vi "at Max velocity.vi"(8 "error in (no error) 2":errorcluster, 9 "Previous Velocity 2":i32, 10 "Previous Velocity":i32) -> (0 "error out 2":errorcluster, 1 "New Velocity 2":i32, 2 "New Velocity":i32, 3 "Max Velocity":bool)   [LabVIEW 2017]
uses:
  Public/Documents/Cross The Road Electronics/Phoenix-LabVIEW/Motor Controller/Get/CTRE_Phoenix_MotorController_GetSelectedSensorData.vi
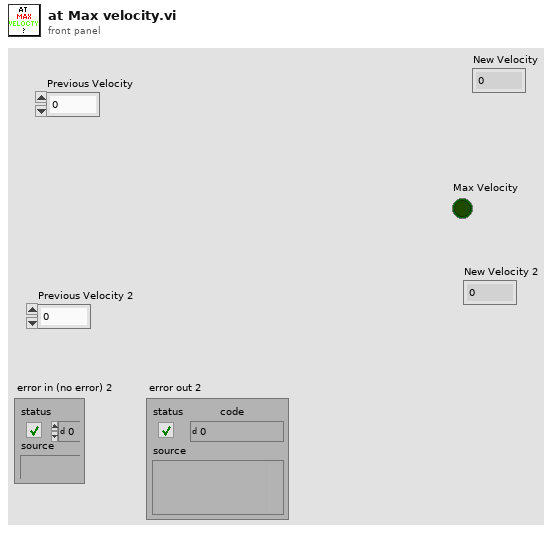
[diagram p1: front panel]
types:
  T1 = typedef "WPI_MotorControlDeviceRef.ctl" = cluster{"DeviceStatus":errorcluster, "Type":T2, "PWM":cluster{"PWM Channel":T3, "DeadBand":T4}, "CAN":cluster{"Device Number":u8, "SetOutput VI Ref":variant, "GetOutput VI Ref":variant, "Enable VI Ref":variant, "Disable VI Ref":variant, "Data":variant}, "Invert":bool, "DIO PWM":cluster{"PWM \"Enable\" Channel":T3, "DIOChannel":T5, "PWM Rate":dbl}}
  T2 = typedef "WPI_MotorControlType.ctl" = enum16{"PWM", "CAN", "DIO PWM"}
  T3 = typedef "FPGA_DIOPWMChannel.ctl" = enum8{"PWM 0", "PWM 1", "PWM 2", "PWM 3", "PWM 4", "PWM 5", "PWM 6", "PWM 7", "PWM 8", "PWM 9", "PWM MXP 0", "PWM MXP 1", "PWM MXP 2", "PWM MXP 3", "PWM MXP 4", "PWM MXP 5", "PWM MXP 6", "PWM MXP 7", "PWM MXP 8", "PWM MXP 9", "Invalid"}
  T4 = typedef "WPI_PWMDeadband.ctl" = cluster{"Name":string, "maxPositivePwm":i32, "minPositivePwm":i32, "centerPwm":i32, "maxNegativePwm":i32, "minNegativePwm":i32, "angularRange":u16}
  T5 = typedef "FPGA_DIOChannel.ctl" = enum8{"DIO 0", "DIO 1", "DIO 2", "DIO 3", "DIO 4", "DIO 5", "DIO 6", "DIO 7", "DIO 8", "DIO 9", "DIO MXP 0", "DIO MXP 1", "DIO MXP 2", "DIO MXP 3", "DIO MXP 4", "DIO MXP 5", "DIO MXP 6", "DIO MXP 7", "DIO MXP 8", "DIO MXP 9", "DIO MXP 10", "DIO MXP 11", "DIO MXP 12", "DIO MXP 13", "DIO MXP 14", "DIO MXP 15", "SPI Port CS1", "SPI Port CS2", "SPI Port CS3", "SPI Port MISO", "SPI Port MOSI", "Invalid"}
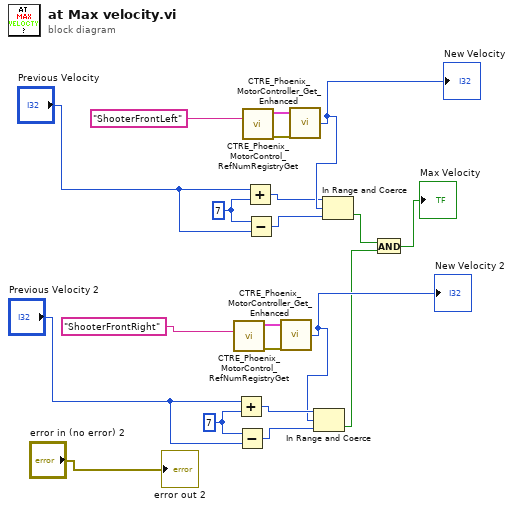
[diagram p0: block diagram]
diagram:
  w11 = 7
  w15 = 7
  n1 = call "CTRE_Phoenix_MotorControl_RefNumRegistryGet.vi"("refnum name"="ShooterFrontRight") -> ("error out"=w6:errorcluster, "PhoenixMotorControlDevRef"=w7:T1)  [unwired: 9 in]
  n2 = Add(x="Previous Velocity 2", y=w11) -> (x+y=w9:i32)
  n3 = Subtract(x=w11, y="Previous Velocity 2") -> (x-y=w10:i32)
  n4 = call "CTRE_Phoenix_MotorControl_RefNumRegistryGet.vi"("refnum name"="ShooterFrontLeft") -> ("error out"=w20:errorcluster, "PhoenixMotorControlDevRef"=w19:T1)  [unwired: 9 in]
  n5 = Add(x="Previous Velocity", y=w15) -> (x+y=w17:i32)
  n6 = Subtract(x=w15, y="Previous Velocity") -> (x-y=w16:i32)
  n7 = call-poly "CTRE_Phoenix_MotorController_Get_Enhanced.vi"("PhoenixMotorControlDevRef"=w7, "error in"=w6) -> ("Velocity (Raw Sensor Units per 100 ms)"=w8:i32)  [unwired: 10 in, 3 out]
  "New Velocity 2" <- w8
  n8 = call-poly "CTRE_Phoenix_MotorController_Get_Enhanced.vi"("PhoenixMotorControlDevRef"=w19, "error in"=w20) -> ("Velocity (Raw Sensor Units per 100 ms)"=w18:i32)  [unwired: 10 in, 3 out]
  "New Velocity" <- w18
  n9 = In Range and Coerce(upper limit=w9, x=w8, lower limit=w10) -> (In Range?=w4:bool)  [unwired: 1 out]
  n10 = In Range and Coerce(upper limit=w17, x=w18, lower limit=w16) -> (In Range?=w5:bool)  [unwired: 1 out]
  n11 = And(x=w5, y=w4) -> (x .and. y?=→"Max Velocity":bool)
  "error out 2" <- "error in (no error) 2"
